vi "Read Results.vi"(8 "error in (no error)":errorcluster, 11 "Project Builder in":refnum<class "Project Builder.lvclass">) -> (0 "error out":errorcluster, 2 "Results":refnum<class "Report Data.lvclass">[](array[class]), 3 "Project Builder out":refnum<class "Project Builder.lvclass">)   [LabVIEW 2019, in "ProjectBuilder.lvlib" / "Project Builder.lvclass"]
doc: "Read 'Result array' from the private data."
uses:
  Project Builder.lvclass
  Data/Report Data/Report Data.lvclass
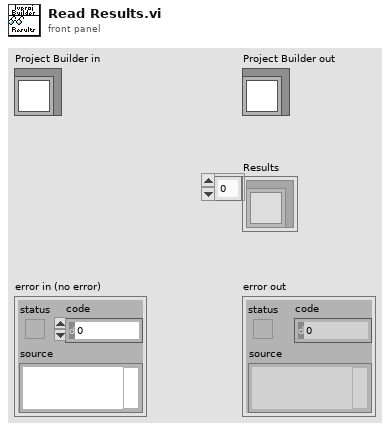
[diagram p1: front panel]
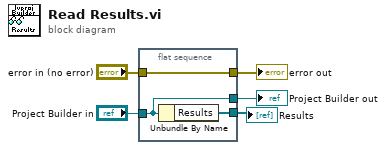
[diagram p0: block diagram]
diagram:
  n1 = flat-sequence {
    tunnel: "error in (no error)" -> [w8]
    tunnel: [w8] -> w4
    tunnel: "Project Builder in" -> [w7]
    tunnel: [w7] -> w2
    tunnel: [w6] -> w1
    frame #0 {
      n2 = Unbundle By Name(w7) -> ("Results"=w6:refnum<class "Report Data.lvclass">[])
    }
  }
  "error out" <- w4
  "Project Builder out" <- w2
  "Results" <- w1
